vi "Start Channels.vi"(8 "error in (no error)":errorcluster, 11 "Performanced XNET CAN Signal Logger in":refnum<class "Performanced XNET CAN Signal Logger.lvclass">) -> (0 "error out":errorcluster, 3 "Performanced XNET CAN Signal Logger out":refnum<class "Performanced XNET CAN Signal Logger.lvclass">)   [LabVIEW 2021, in "Performanced XNET CAN Signal Logger.lvlib" / "Performanced XNET CAN Signal Logger.lvclass"]
uses:
  Performanced XNET CAN Signal Logger.lvclass
  Performanced XNET CAN Signal Logger.lvclass/Performanced XNET CAN Signal Logger.ctl
  XNET-CAN-Signal-Logger.lvlib
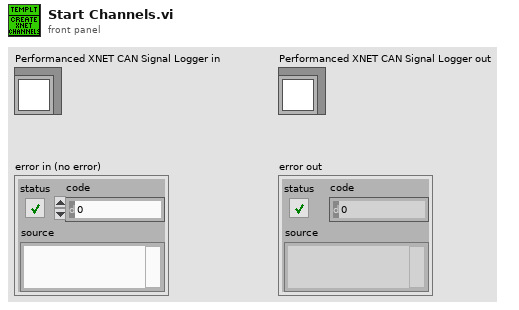
[diagram p1: front panel]
types:
  T1 = typedef "XNET-CAN-Signal-Logger.lvlib/Def-CAN Port Configuration.ctl" = cluster{"CAN Interface":refnum<k21>, "XNET Cluster":refnum<k21>, "#Signals":i32, "Sample Rate (Hz)":dbl}
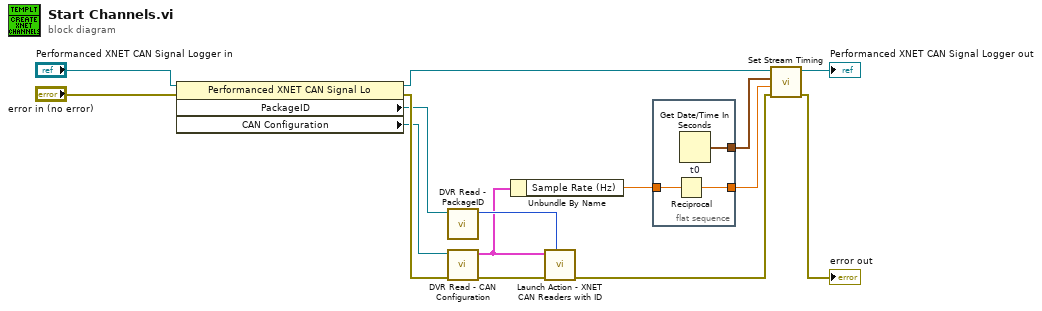
[diagram p0: block diagram]
diagram:
  n1 = property class="Performanced XNET CAN Signal Lo"(reference="Performanced XNET CAN Signal Logger in", error in="error in (no error)") -> (reference out=w6:refnum<class "Performanced XNET CAN Signal Logger.lvclass">, error out=w12:errorcluster, "PackageID"=w9:refnum<data-value>, "CAN Configuration"=w11:refnum<data-value>)
  n2 = call "DVR Read - PackageID.vi"("Data Value Reference in"=w9) -> ("PackageID"=w10:i32)  [unwired: 10 in]
  n3 = call "DVR Read - CAN Configuration.vi"("Data Value Reference in"=w11) -> ("CAN Port Configuration"=w2:T1)  [unwired: 10 in]
  n4 = Unbundle By Name(w2) -> ("Sample Rate (Hz)"=w1:dbl)
  n5 = call "Launch Action - XNET CAN Readers with ID.vi"("PackageID"=w10, "error in (no error)"=w12, "CAN Configuration"=w2) -> ("error out"=w4:errorcluster)  [unwired: 8 in]
  n6 = flat-sequence {
    tunnel: [w17] -> w7
    tunnel: [w16] -> w8
    tunnel: w1 -> [w15]
    frame #0 {
      n7 = Reciprocal(x=w15) -> (1/x=w16:dbl)
      n8 = Get Date/Time In Seconds "t0"() -> (seconds since 1Jan1904=w17:timestamp)
    }
  }
  n9 = call-dynamic "Set Stream Timing.vi"("error in (no error)"=w4, "dt(sec)"=w8, "Start Time"=w7, "Plugin in"=w6) -> ("error out"=→"error out":errorcluster, "Plugin out"=→"Performanced XNET CAN Signal Logger out":refnum<class "Performanced XNET CAN Signal Logger.lvclass">)  [unwired: 6 in]
